vi "wait for good link.vi"(8 "error in":errorcluster, 9 "timeout s(10)":u32=10, 10 "port id":u32, 11 "InstrumentHandle_board in":u32) -> (0 "error out":errorcluster, 1 "timed out":bool, 2 "good link":bool, 3 "InstrumentHandle_board out":u32)   [LabVIEW 2020]
uses:
  src/AIM664LV.lvlib
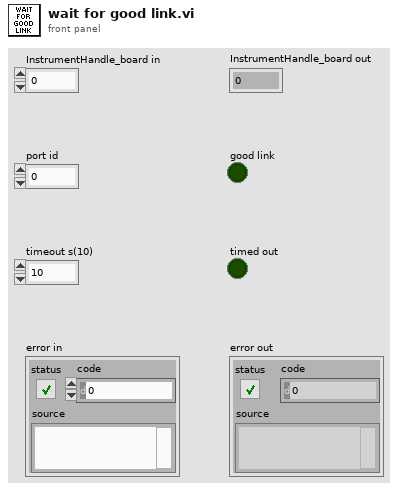
[diagram p1: front panel]
types:
  T1 = typedef "AIM664LV.lvlib/port_configuration.ctl" = u32
  T2 = typedef "AIM664LV.lvlib/port_speed.ctl" = u32
  T3 = typedef "AIM664LV.lvlib/port_condition.ctl" = u32
  T4 = typedef "AIM664LV.lvlib/expert_mode.ctl" = u32
  T5 = cluster{"PortConfig":T1[], "PortSpeed":T2[], "PortUsed":u32[], "PortGoodLink":T3[], "ExpertMode":T4[], "GlobalMemFree":u32, "SharedMemFree":u32, "RxVeriMode":u32}
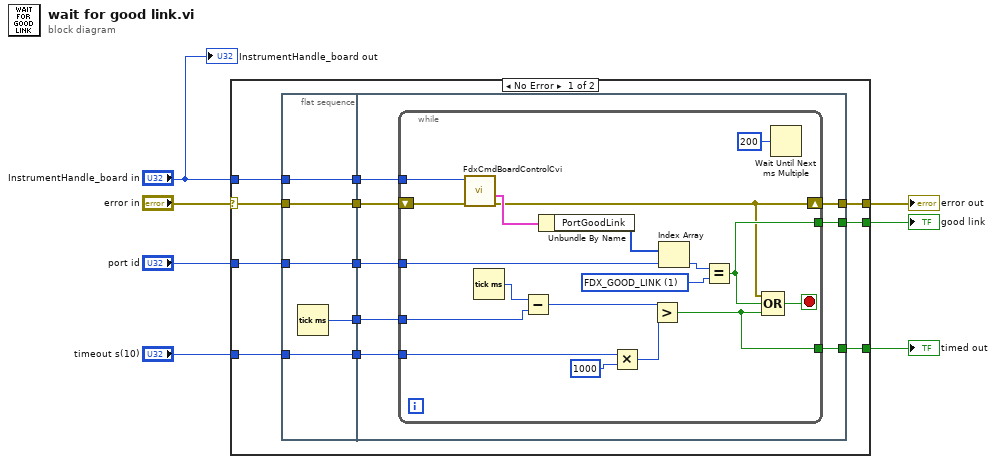
[diagram p0: block diagram]
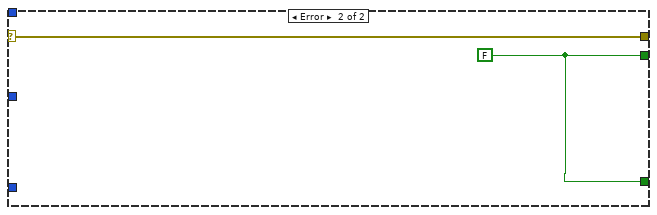
[diagram p2: hidden frame]
diagram:
  n1 = case shown="No Error" "error in" {
    selector: "error in" -> [w14 w52]
    tunnel: "timeout s(10)" -> [w19 _]
    tunnel: "port id" -> [w18 _]
    tunnel: [w17 w51] -> w4
    tunnel: [w16 w51] -> w5
    tunnel: [w15 w52] -> w6
    tunnel: "InstrumentHandle_board in" -> [w13 _]
    frame No Error {
      n2 = flat-sequence {
        tunnel: w13 -> [w21]
        tunnel: w14 -> [w22]
        tunnel: w18 -> [w23]
        tunnel: w19 -> [w24]
        tunnel: [w24] -> w12
        tunnel: [w23] -> w11
        tunnel: [w22] -> w10
        tunnel: [w21] -> w9
        tunnel: [w20] -> w8
        tunnel: [w30] -> w17
        tunnel: [w29] -> w16
        tunnel: [w28] -> w15
        tunnel: w12 -> [w32]
        tunnel: w11 -> [w31]
        tunnel: w10 -> [w27]
        tunnel: w9 -> [w26]
        tunnel: w8 -> [w25]
        frame #0 {
          n3 = Tick Count (ms)() -> (millisecond timer value=w20:u32)
        }
        frame #1 {
          n4 = while {
            tunnel: w32 -> [w48]
            tunnel: w31 -> [w42]
            tunnel: [w40] -> w30
            tunnel: [w37] -> w29
            shift-right: [w36] -> w28
            shift-left: w27 -> [w35]
            tunnel: w26 -> [w34]
            tunnel: w25 -> [w33]
            stop <- w41 stop-if-true
            w38 = u32 1 items=["FDX_NO_LINK", "FDX_GOOD_LINK"]
            n5 = call "FdxCmdBoardControlCvi.vi"("error in"=w35, "InstrumentHandle_board in"=w34) -> ("error out"=w36:errorcluster, "Board Control Out"=w50:T5)  [unwired: 7 in, 1 out]
            n6 = Tick Count (ms)() -> (millisecond timer value=w46:u32)
            n7 = Subtract(x=w46, y=w33) -> (x-y=w44:u32)
            n8 = Unbundle By Name(w50) -> ("PortGoodLink"=w49:T3[])
            n9 = Multiply(x=w48, y=u32 1000) -> (x*y=w43:u32)
            n10 = Greater?(x=w44, y=w43) -> (0:w40:bool)
            n11 = Index Array(array=w49, index=w42) -> (element=w39:T3)
            n12 = Equal?(x=w39, y=w38) -> (x = y?=w37:bool)
            n13 = Compound Arithmetic op=OR(w36, w37, w40) -> (w41:bool)
            n14 = Wait Until Next ms Multiple(millisecond multiple=u32 200) -> ()  [unwired: 1 out]
          }
        }
      }
    }
    frame Error {
      w51 = FALSE
    }
  }
  "error out" <- w6
  "good link" <- w5
  "timed out" <- w4
  "InstrumentHandle_board out" <- "InstrumentHandle_board in"
